vi "DB Variant To Data_ErrorHandler.vi"(0 "data in":variant, 11 "error in (no error)":errorcluster, 12 "initial error in":errorcluster) -> (4 "data out":variant, 15 "error out":errorcluster={"status"=FALSE, "code"=0, "source"="0"})   [LabVIEW 2013, in "NI_DB Variant To Data Support.lvlib"]
uses:
  <vilib>/addons/database/_DB Variant To Data/NI_DB Variant To Data Support.lvlib
panel:
  # "terminals:\ndata in = 0\ndata out = 4\nerror in = 11\nerror out = 15\ninitial error in = 12"
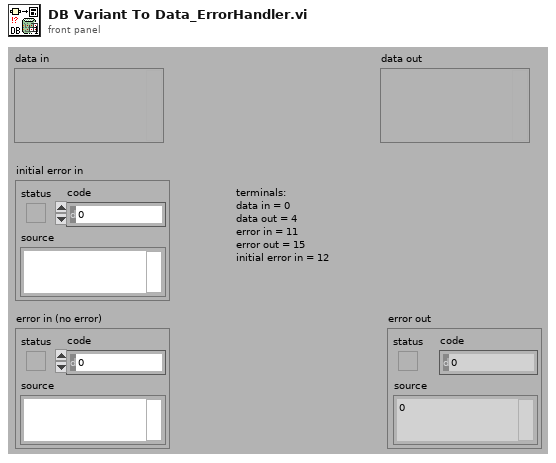
[diagram p1: front panel]
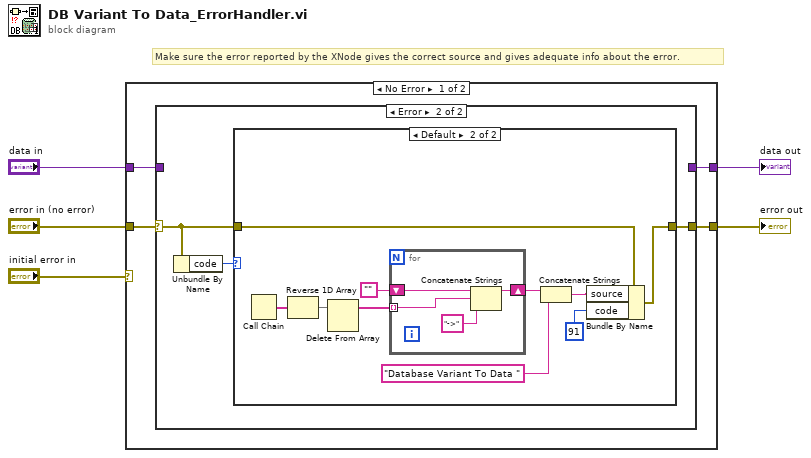
[diagram p0: block diagram]
diagram:
  # "Make sure the error reported by the XNode gives the correct source and gives adequate info about the error."
  n1 = case shown="No Error" "initial error in" {
    selector: "initial error in" -> [_ w30]
    tunnel: [w9 w30] -> w4
    tunnel: "data in" -> [w7 w29]
    tunnel: [w8 w29] -> w2
    tunnel: "error in (no error)" -> [w6 _]
    frame No Error {
      n2 = case shown="Error" w6 {
        selector: w6 -> [w10 w12]
        tunnel: [w10 w14] -> w9
        tunnel: [w11 _] -> w8
        tunnel: w7 -> [w11 _]
        frame No Error {
          # "pass through warnings"
        }
        frame Error {
          n3 = Unbundle By Name(w12) -> ("code"=w13:i32)
          n4 = case shown="Default" w13 {
            tunnel: [_ w24] -> w14
            tunnel: w12 -> [_ w15]
            frame -2147467261 {
              # "Variant To Data returns -2147467261 if the variant input is NULL.  We want to clear the error and pass back default data."
            }
            frame Default {
              n5 = Call Chain() -> (call chain=w21:string[])
              n6 = Reverse 1D Array(array=w21) -> (reversed array=w20:string[])
              n7 = Delete From Array(array=w20) -> (array with subset deleted=w19:string[])  [unwired: 2 in, 1 out]
              n8 = for {
                tunnel: w19 -> [w27] mode=indexing
                shift-right: [w28] -> w18
                shift-left: "" -> [w26]
                n9 = Concatenate Strings(w26, w27, "->" ("string")) -> (w28:string)
              }
              n10 = Concatenate Strings(w18, "Database Variant To Data " ("source")) -> (w22:string)
              n11 = Bundle By Name(cluster=w15, "source"=w22, "code"=91) -> (w24:errorcluster)
            }
          }
        }
      }
    }
    frame Error {
    }
  }
  "error out" <- w4
  "data out" <- w2
